vi "car_battery.vi"(1 "read buffer":string) -> (0 "输出簇":cluster{"C_Battery":dbl, "D_Battery\n":dbl})   [LabVIEW 2014]
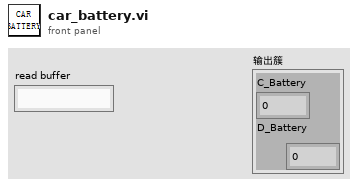
[diagram p1: front panel]
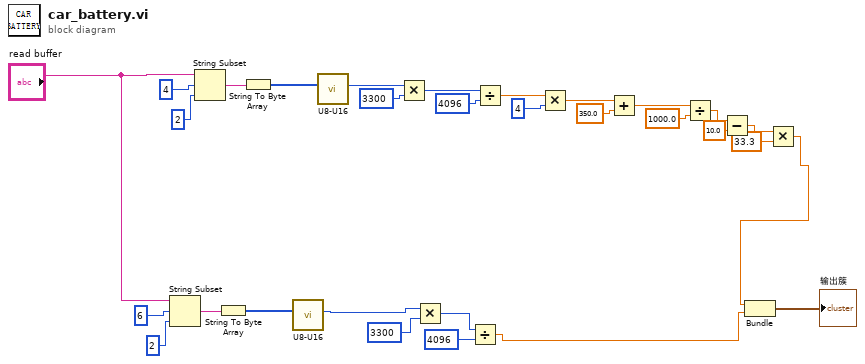
[diagram p0: block diagram]
diagram:
  n1 = String Subset(string="read buffer", offset (0)=6 ("长度（剩余）"), length (rest)=2 ("长度（剩余）")) -> (substring=w30:string)
  n2 = String Subset(string="read buffer", offset (0)=4 ("长度（剩余）"), length (rest)=2 ("长度（剩余）")) -> (substring=w26:string)
  n3 = String To Byte Array(string=w30) -> (unsigned byte array=w27:u8[])
  n4 = String To Byte Array(string=w26) -> (unsigned byte array=w23:u8[])
  n5 = call "U8-U16.vi"("数组"=w27) -> ("16位整型"=w14:u16)  [unwired: 8 in, 1 out]
  n6 = call "U8-U16.vi"("数组"=w23) -> ("16位整型"=w20:u16)  [unwired: 8 in, 1 out]
  n7 = Multiply(x=w20, y=3300) -> (x*y=w13:i32)
  n8 = Multiply(x=w14, y=3300) -> (x*y=w16:i32)
  n9 = Divide(x=w16, y=4096) -> (x/y=w6:dbl)
  n10 = Divide(x=w13, y=4096) -> (x/y=w11:dbl)
  n11 = Multiply(x=w11, y=4) -> (x*y=w10:dbl)
  n12 = Add(x=w10, y=350.0) -> (x+y=w8:dbl)
  n13 = Divide(x=w8, y=1000.0) -> (x/y=w5:dbl)
  n14 = Subtract(x=w5, y=10.0) -> (x-y=w3:dbl)
  n15 = Multiply(x=w3, y=33.3) -> (x*y=w1:dbl)
  n16 = Bundle(w1, w6) -> (→"输出簇":cluster{dbl, dbl})  [unwired: 1 in]
